vi "Subscr.Service Subscriptions.vi"(8 "error in (no error)":errorcluster, 9 "Data":variant, 10 "Name":string, 11 "Subscription in":refnum<class "Subscription.lvclass">) -> (0 "error out":errorcluster, 3 "Subscription out":refnum<class "Subscription.lvclass">)   [LabVIEW 2024, in "EQMF.lvlib" / "Subscription.lvlib" / "Subscription.lvclass"]
uses:
  Subscription.lvclass
  Subscr.Subscription Request Info.ctl
  Queues/Q.Element.ctl
  Subscription.lvclass/Subscription.ctl
  Queues/Queue Utils.lvlib
  Subscription.lvlib
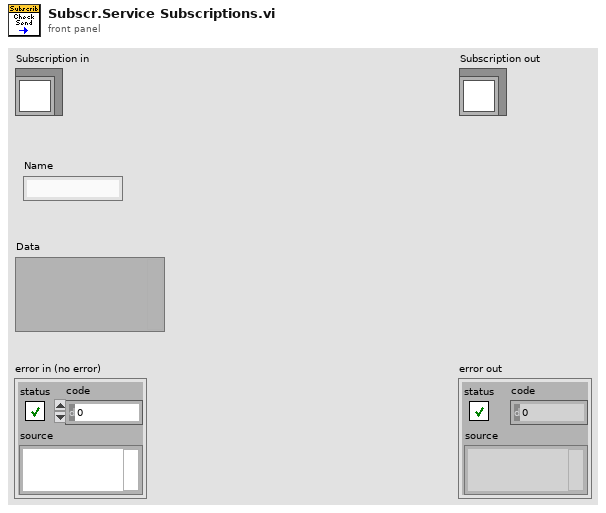
[diagram p1: front panel]
types:
  T1 = typedef "EQMF.lvlib/Subscription.lvlib/Subscr.Subscription Request Info.ctl" = cluster{"Name":string, "Data Q":refnum<queue>, "Data Element":T2}
  T2 = typedef "EQMF.lvlib/Queue Utils.lvlib/Q.Element.ctl" = cluster{"Cmd":string, "Sub":string, "Data1":variant, "Data2":variant}
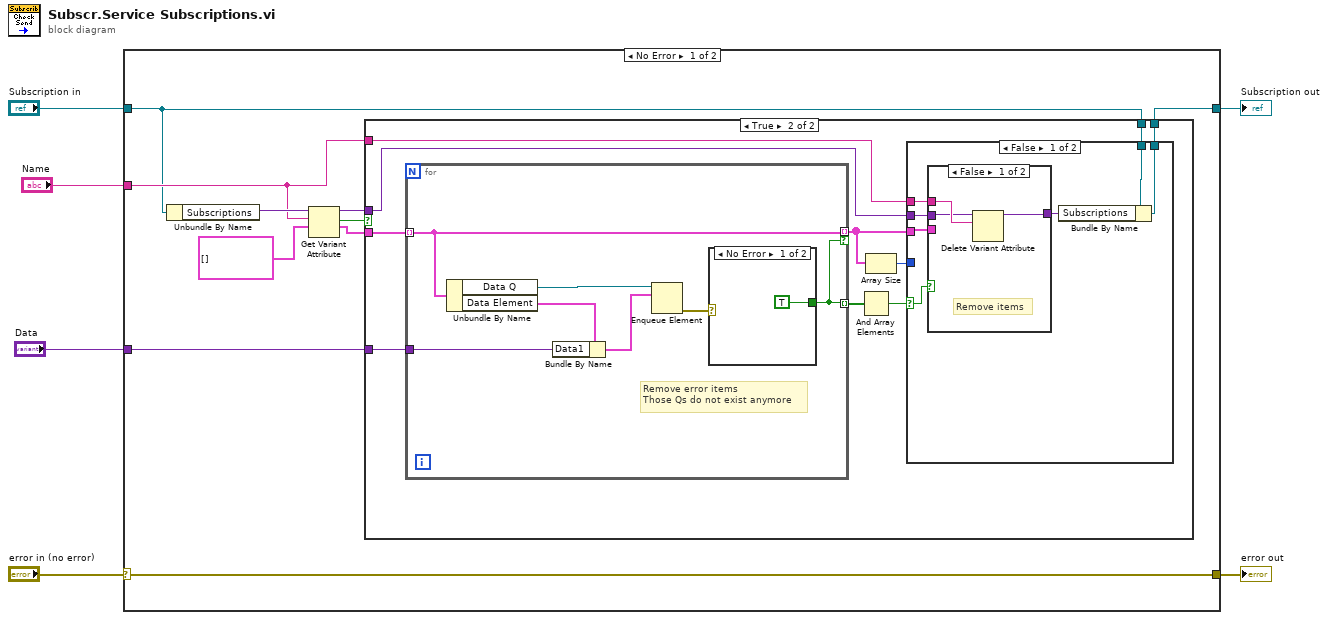
[diagram p0: block diagram]
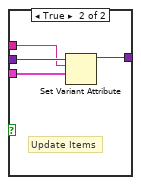
[diagram p3: hidden frame]
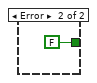
[diagram p5: hidden frame]
diagram:
  n1 = case shown="No Error" "error in (no error)" {
    selector: "error in (no error)" -> [w16 w53]
    tunnel: [w16 w53] -> w5
    tunnel: [w8 w52] -> w3
    tunnel: "Subscription in" -> [w7 w52]
    tunnel: "Data" -> [w11 _]
    tunnel: "Name" -> [w9 _]
    frame No Error {
      n2 = Unbundle By Name(w7) -> ("Subscriptions"=w15:variant)
      n3 = Get Variant Attribute(Variant=w15, name=w9, default value (empty Variant)=T1[] []) -> (duplicate Variant=w10:variant, found=w13:bool, value=w12:T1[])  [unwired: 1 in, 1 out]
      n4 = case shown="True" w13 {
        tunnel: w12 -> [_ w27]
        tunnel: w11 -> [_ w26]
        tunnel: w7 -> [w17 w21]
        tunnel: w10 -> [_ w23]
        tunnel: w9 -> [_ w22]
        tunnel: [w17 w20] -> w8
        frame False {
        }
        frame True {
          n5 = for {
            tunnel: w27 -> [w46] mode=indexing
            tunnel: w26 -> [w45]
            tunnel: [w46] -> w19 mode=indexing if=w43
            tunnel: [w43] -> w25 mode=indexing
            # "Remove error items\nThose Qs do not exist anymore"
            n6 = Unbundle By Name(w46) -> ("Data Q"=w49:refnum<queue>, "Data Element"=w48:T2)
            n7 = Bundle By Name(cluster=w48, "Data1"=w45) -> (w47:T2)
            n8 = Enqueue Element(queue=w49, element=w47) -> (error out=w44:errorcluster)  [unwired: 2 in, 2 out]
            n9 = case shown="No Error" w44 {
              tunnel: [TRUE FALSE] -> w43
              frame No Error {
              }
              frame Error {
              }
            }
          }
          n10 = And Array Elements(Boolean array=w25) -> (logical AND=w24:bool)
          n11 = Array Size(array=w19) -> (size(s)=w18:i32)
          n12 = case shown="False" w24 {
            selector: w24 -> [w28 _]
            tunnel: w19 -> [w32 _]
            tunnel: w23 -> [w34 _]
            tunnel: w22 -> [w33 _]
            tunnel: w21 -> [w31 w42]
            tunnel: [w29 w42] -> w20
            tunnel: w18 -> [_ _]
            frame False {
              n13 = case shown="False" w28 {
                tunnel: w34 -> [w36 w41]
                tunnel: w33 -> [w37 w40]
                tunnel: w32 -> [_ w39]
                tunnel: [w35 w38] -> w30
                frame False {
                  # "Remove items"
                  n14 = Delete Variant Attribute(6:w37, 7:w36) -> (3:w35:variant)  [unwired: 1 in, 2 out]
                }
                frame True {
                  # "Update Items"
                  n15 = Set Variant Attribute(Variant=w41, name=w40, value=w39) -> (Variant out=w38:variant)  [unwired: 1 in, 2 out]
                }
              }
              n16 = Bundle By Name(cluster=w31, "Subscriptions"=w30) -> (w29:refnum<class "Subscription.lvclass">)
            }
            frame True {
              # "No Change"
            }
          }
        }
      }
    }
    frame Error {
    }
  }
  "error out" <- w5
  "Subscription out" <- w3
